vi "writeFile TestID.vi"(8 "TestID":u32, 11 "Path":path=path "C:/Users/Flash/Desktop/LabVIEW/Detector IV/rawtest_log.csv") -> ()   [LabVIEW 2012]
uses:
  <vilib>/Utility/file.llb/Write To Spreadsheet File (I64).vi
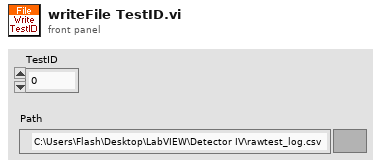
[diagram p1: front panel]
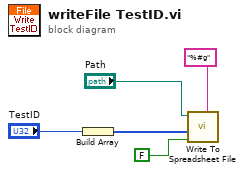
[diagram p0: block diagram]
diagram:
  n1 = Build Array("TestID") -> (w1:u32[])
  n2 = call-poly <vilib>:"Write To Spreadsheet File.vi"("format (%d)"="%#g" ("format (%.3f)"), "append to file? (new file:F)"=FALSE, "1D data"=w1, "file path (dialog if empty)"="Path") -> ()  [unwired: 3 in, 2 out]
